vi "Shut Down Async Loops.vi"(0 "VI Refs":refnum<vi>[](array[refnum]), 11 "error in (no error)":errorcluster) -> (15 "error out":errorcluster)   [LabVIEW 2011, in "AIT 1553 Custom Device.lvlib"]
uses:
  AIT 1553 Custom Device.lvlib
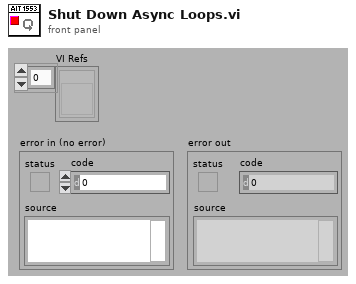
[diagram p1: front panel]
types:
  T1 = enum32{"Bad", "Idle", "Run top level", "Running"}
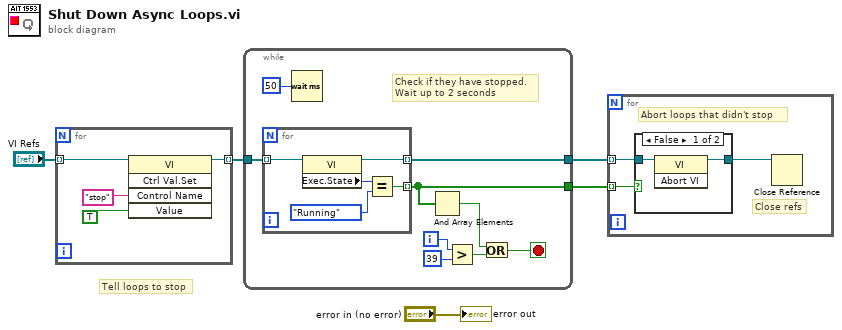
[diagram p0: block diagram]
diagram:
  # "Tell loops to stop"
  n1 = for {
    tunnel: "VI Refs" -> [w9] mode=indexing
    tunnel: [w7] -> w4 mode=indexing
    n2 = invoke class="VI" method="Ctrl Val.Set"(reference=w9, "Control Name"="stop", "Value"=TRUE ("force destroy? (F)")) -> (reference out=w7:refnum<vi>)  [unwired: 2 in, 4 out]
  }
  n3 = while {
    tunnel: w4 -> [w17]
    tunnel: [w16] -> w2
    tunnel: [w11] -> w3
    i -> [w14]
    stop <- w15 stop-if-true
    # "Check if they have stopped.\nWait up to 2 seconds"
    n4 = for {
      tunnel: w17 -> [w23] mode=indexing
      tunnel: [w19] -> w11 mode=indexing
      tunnel: [w22] -> w16 mode=indexing
      n5 = property class="VI"(reference=w23) -> (reference out=w22:refnum<vi>, "Exec.State"=w21:T1)  [unwired: 1 in, 1 out]
      n6 = Equal?(x=w21, y=T1."Running") -> (x = y?=w19:bool)
    }
    n7 = Wait (ms)(milliseconds to wait=u32 50) -> ()  [unwired: 1 out]
    n8 = And Array Elements(Boolean array=w11) -> (logical AND=w10:bool)
    n9 = Greater?(x=w14, y=39) -> (0:w12:bool)
    n10 = Or(x=w10, y=w12) -> (x .or. y?=w15:bool)
  }
  n11 = for {
    tunnel: w2 -> [w26] mode=indexing
    tunnel: w3 -> [w25] mode=indexing
    # "Close refs"
    # "Abort loops that didn't stop"
    n12 = case shown="False" w25 {
      tunnel: w26 -> [w28 w29]
      tunnel: [w27 w29] -> w24
      frame False {
        n13 = invoke class="VI" method="Abort VI"(reference=w28) -> (reference out=w27:refnum<vi>)  [unwired: 2 in, 2 out]
      }
      frame True {
      }
    }
    n14 = Close Reference(reference=w24) -> ()  [unwired: 1 in, 1 out]
  }
  "error out" <- "error in (no error)"
